vi "Set Page Size.vi"(0 "PDF Report IN":T21(xcontrol), 2 "Page setup":T22={"Page Size"=1, "Orientation"=enum."Portrait", "Custom Layout"={"Width"=0.0, "Height"=0.0}, "Margins"={"Left"=25.0, "Right"=25.0, "Top"=25.0, "Bottom"=25.0}} {"Page Size" items=["Custom", "LETTER", "NOTE", "LEGAL", "TABLOID", "EXECUTIVE", "POSTCARD", "A0", "A1", "A2", "A3", "A4", "A5", "A6", "A7", "A8", "A9", "A10", "B0", "B1", "B2", "B3", "B4", "B5", "B6", "B7", "B8", "B9", "B10", "ARCH_E", "ARCH_D", "ARCH_C", "ARCH_B", "ARCH_A", "FLSA", "FLSE", "HALFLETTER", "_11X17", "ID_1", "ID_2", "ID_3", "LEDGER", "CROWN_QUARTO", "LARGE_CROWN_QUARTO", "DEMY_QUARTO", "ROYAL_QUARTO", "CROWN_OCTAVO", "LARGE_CROWN_OCTAVO", "DEMY_OCTAVO", "ROYAL_OCTAVO", "SMALL_PAPERBACK", "PENGUIN_SMALL_PAPERBACK", "PENGUIN_LARGE_PAPERBACK"]}, 11 "error in (no error)":errorcluster) -> (4 "PDF Report OUT":T21(xcontrol), 15 "error OUT":errorcluster)   [LabVIEW 2013]
doc: "Creates a page break within the PDF report and change the layout of the new page:\n- Page size;\n- Orientation;\n- Margins (mm or in);\n- Custom layout (if Page size = custom, mm or in);\n\nMinimum page size: 3 points x 3 points (1.06 mm x 1.06 mm or 0.042 in x 0.042 in)\nMaximum page size: 14400 points x 14400 points (5.08 m x 5.08 m or 200 in x 200 in)\n\n<B>FRANÇAIS</B>\nAjoute un saut de page dans le rapport PDF et change les caractéristiques de la nouvelle page :\n- Format de la page;\n- Orientation;\n- Marges (mm or in);\n- Format personnalisé (si Page size = custom, mm ou in).\n\nDimensions minimales d'une page: 3 points x 3 points (1.06 mm x 1.06 mm or 0.042 in x 0.042 in).\nDimensions maximales d'une page: 14400 points x 14400 points (5.08 m x 5.08 m or 200 in x 200 in).\n\nVersion 1.0\nDeveloped by Jean-Marc Simard\nCopyright © 2010, Exaprom Inc.\nAll rights reserved.\nLicense: BSD\n\nWith iTextSharp 4.1.6 (http://itextsharp.sourceforge.net)\nunder Mozilla Public License Version 1.1\n(http://www.mozilla.org/MPL/MPL-1.1.html)"
uses:
  Controls/Page setup.ctl
  Controls/Page size.ctl
  Controls/Page Orientation.ctl
  Controls/Page Layout Custom.ctl
  Controls/Page margins.ctl
  Controls/PDF Report Xcontrol/PDF Report.xctl
  C:/Users/MaxCorp/Documents/GitHub/TopView/DLL/itextsharp.dll
  DLL/itextsharp.dll
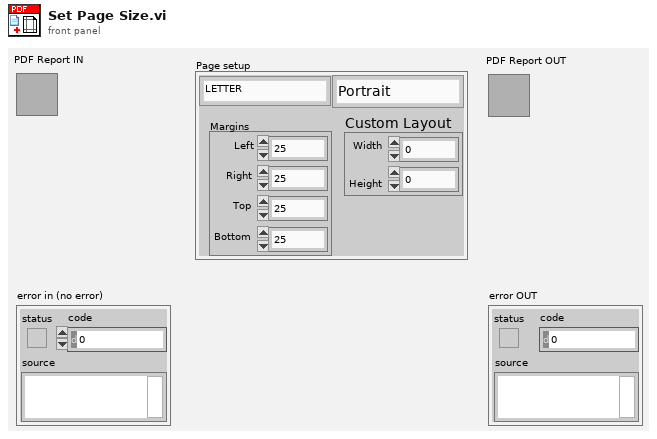
[diagram p1: front panel]
types:
  T1 = typedef "Font cluster.ctl" = cluster{"Name":string, "Size":T2, "Color":T3, "Style":cluster{"Bold":bool, "Italic":bool, "Underline":bool, "Strikeout":bool}}
  T2 = typedef "Font size.ctl" = sgl
  T3 = typedef "Font color.ctl" = u32
  T4 = typedef "Unit.ctl" = enum16{"inch", "mm"}
  T5 = typedef "Paragraphe cluster.ctl" = cluster{" Aligment":T6, "Line spacing":T7}
  T6 = typedef "Texte alignement.ctl" = enum16{"Select", "CENTER", "JUSTIFY", "LEFT", "RIGHT"}
  T7 = typedef "Line spacing.ctl" = enum16{"Select", "1.0", "1.5", "2.0"}
  T8 = typedef "Page dimensions.ctl" = cluster{"Start at page":i32, "Orientation":T9, "widht":sgl, "height":sgl, "Margin left":sgl, "Margin right":sgl, "Margin top":sgl, "Margin bottom":sgl}
  T9 = typedef "Page Orientation.ctl" = enum16{"Portrait", "Landscape"}
  T10 = typedef "Image or Table Caption.ctl" = cluster{"Caption":string, "Separator":string, "Position":enum16{"Above", "Below"}}
  T11 = typedef "Header Footer [ ].ctl" = T12[]
  T12 = typedef "Header Footer cluster.ctl" = cluster{"Start page":i32, "Type":T13, "Alignment":T14, "Vertical Alignement":T15, "Image (%)":sgl, "Page #":T16, "Text":string, "Path":string, "Font":T1, "Font refnum":refnum<k24>, "Line":cluster{"Line":T17, "Thickness (points)":sgl, "Colour":T3}}
  T13 = typedef "Header Footer Type.ctl" = enum16{"Select", "Text", "Text + hyperlink", "Page number", "Image", "Image + hyperlink"}
  T14 = typedef "Header footer horiz alignment.ctl" = enum16{"Left", "Center", "Right"}
  T15 = typedef "Cell Vertical alignment.ctl" = enum16{"TOP", "MIDDLE", "BOTTOM"}
  T16 = typedef "Page number.ctl" = cluster{"Text 1":string, "Text 2":string, "Text 3":string}
  T17 = typedef "Header Footer Line.ctl" = enum16{"No line", "Horizontal line"}
  T18 = typedef "Watermark cluster2.ctl" = cluster{"Show? (F)":bool, "Type":enum16{"Image", "Text"}, "Opacity (%)":sgl, "Rotate(°)":sgl, "Position":cluster{"Position":T19, "X":sgl, "Y":sgl}, "Image path":path, "Scaled(%)":sgl, "Image refnum":refnum<k24>, "Text":string, "Font":cluster{"Name":string, "Size":T2, "Color":T3}, "Font refnum":refnum<k24>, "Alignment":T14, "Automatic":bool}
  T19 = typedef "Watermark Position.ctl" = enum16{"Absolute", "Center (page)", "Center (text section)"}
  T20 = typedef "System Fonts.ctl" = cluster{"Font name [ ]":string[], "Font and file names [ ]":cluster{"Font name":string, "File name":string}[]}
  T21 = cluster{"Document":refnum<k24>, "Writer":refnum<k24>, "Default Font":refnum<k24>, "Default Font cluster":T1, "Path":path, "Unit (default = mm)":T4, "Paragraphe cluster":T5, "Pages dimensions [ ]":T8[], "Captions":cluster{"Image":T10, "Image counter":u16, "Table":T10, "Table counter":u16, "Font":T1}, "Header":T11, "Footer":T11, "Watermark ":T18, "Actual VI name":string, "System Fonts":T20}
  T22 = typedef "Page setup.ctl" = cluster{"Page Size":T23, "Orientation":T9, "Custom Layout":T24, "Margins":T25}
  T23 = typedef "Page size.ctl" = i32
  T24 = typedef "Page Layout Custom.ctl" = cluster{"Width":sgl, "Height":sgl}
  T25 = typedef "Page margins.ctl" = cluster{"Left":sgl, "Right":sgl, "Top":sgl, "Bottom":sgl}
  T26 = cluster{"PageNumber":i32, "Orientation":T9, "Width":sgl, "Height":sgl, "LeftMargin":sgl, "RightMargin":sgl, "TopMargin":sgl, "BottomMargin":sgl}
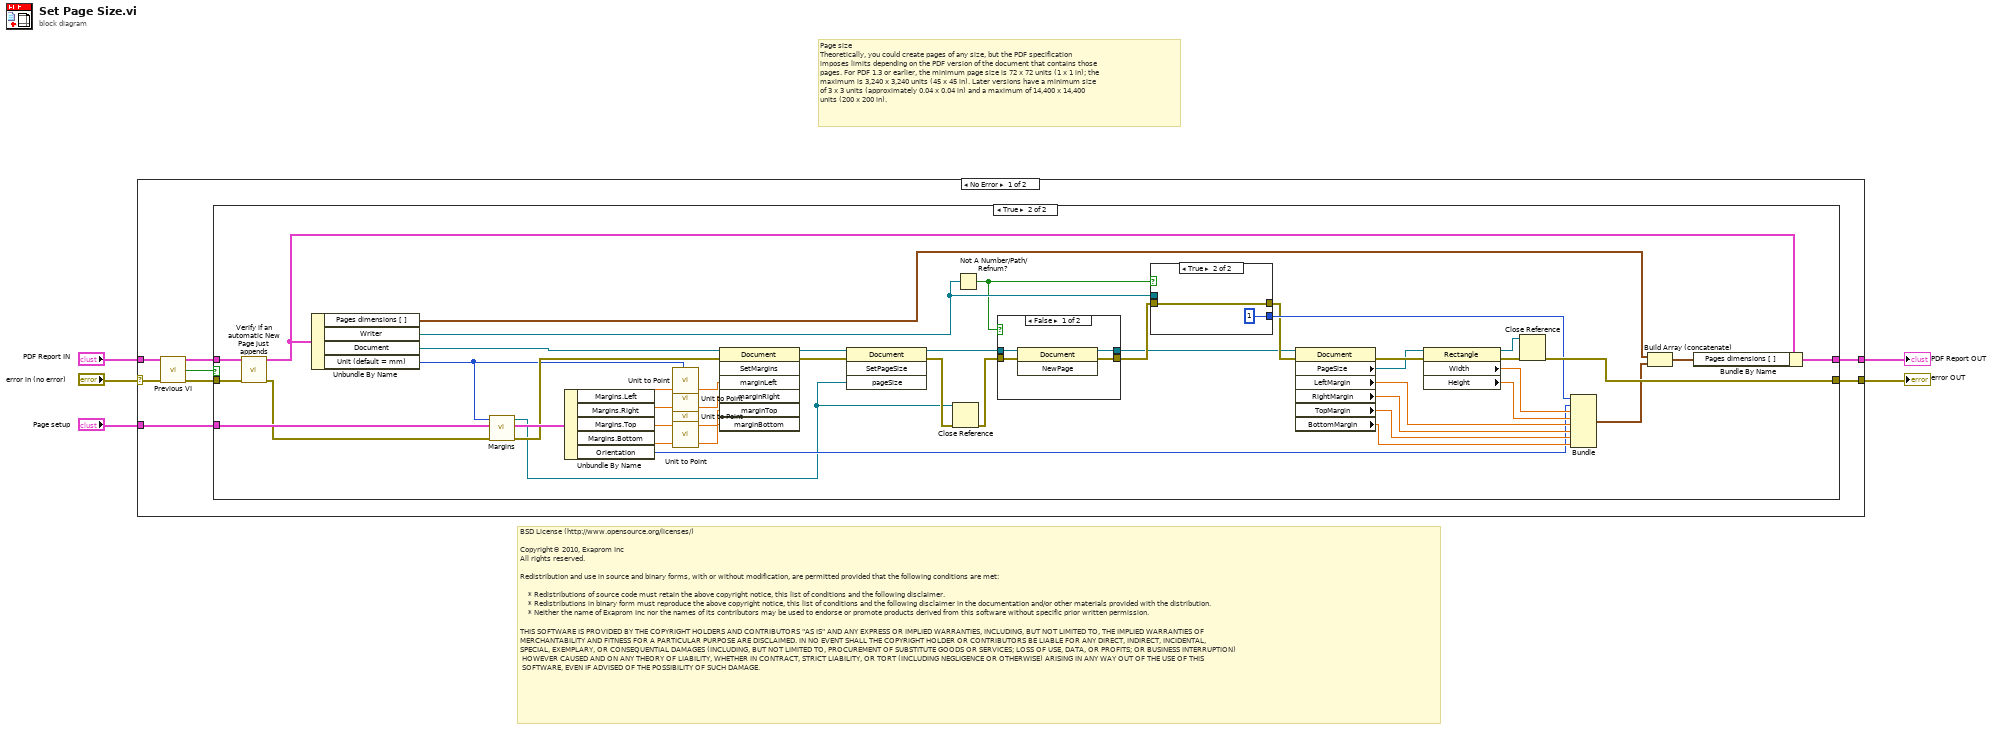
[diagram p0: block diagram]
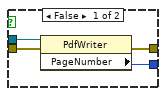
[diagram p4: hidden frame]
diagram:
  # "Page size\nTheoretically, you could create pages of any size, but the PDF specification\nimposes limits depending on the PDF version of the document that contains those\npages. For PDF 1.3 or earlier, the minimum page size is 72 x 72 units (1 x 1 in); the\nmaximum is 3,240 x 3,240 units (45 x 45 in). Later versions have a minimum size\nof 3 x 3 units (approximately 0.04 x 0.04 in) and a maximum of 14,400 x 14,400\nunits (200 x 200 in)."
  # "BSD License (http://www.opensource.org/licenses/)\n\nCopyright© 2010, Exaprom Inc\nAll rights reserved.\n\nRedistribution and use in source and binary forms, with or without modification, are permitted provided that the following conditions are met:\n\n    * Redistributions of source code must retain the above copyright notice, this list of conditions and the following disclaimer.\n    * Redistributions in binary form must reproduce the above copyright notice, this list of conditions and the following disclaimer in the documentation and/or other materials provided with the distribution.\n    * Neither the name of Exaprom Inc nor the names of its contributors may be used to endorse or promote products derived from this software without specific prior written permission.\n\nTHIS SOFTWARE IS PROVIDED BY THE COPYRIGHT HOLDERS AND CONTRIBUTORS \"AS IS\" AND ANY EXPRESS OR IMPLIED WARRANTIES, INCLUDING, BUT NOT LIMITED TO, THE IMPLIED WARRANTIES OF \nMERCHANTABILITY AND FITNESS FOR A PARTICULAR PURPOSE ARE DISCLAIMED. IN NO EVENT SHALL THE COPYRIGHT HOLDER OR CONTRIBUTORS BE LIABLE FOR ANY DIRECT, INDIRECT, INCIDENTAL,\nSPECIAL, EXEMPLARY, OR CONSEQUENTIAL DAMAGES (INCLUDING, BUT NOT LIMITED TO, PROCUREMENT OF SUBSTITUTE GOODS OR SERVICES; LOSS OF USE, DATA, OR PROFITS; OR BUSINESS INTERRUPTION)\n HOWEVER CAUSED AND ON ANY THEORY OF LIABILITY, WHETHER IN CONTRACT, STRICT LIABILITY, OR TORT (INCLUDING NEGLIGENCE OR OTHERWISE) ARISING IN ANY WAY OUT OF THE USE OF THIS\n SOFTWARE, EVEN IF ADVISED OF THE POSSIBILITY OF SUCH DAMAGE."
  n1 = case shown="No Error" "error in (no error)" {
    selector: "error in (no error)" -> [w9 w74]
    tunnel: [w11 w74] -> w3
    tunnel: "Page setup" -> [w6 _]
    tunnel: [w13 w73] -> w2
    tunnel: "PDF Report IN" -> [w12 w73]
    frame No Error {
      n2 = call "Previous VI.vi"("PDF Report IN"=w12, "error in (no error)"=w9) -> ("PDF Report OUT"=w10:T21, "Execute Actual VI"=w8:bool, "error out"=w7:errorcluster)  [unwired: 11 out]
      n3 = case shown="True" w8 {
        tunnel: w6 -> [_ w60]
        tunnel: [w14 w44] -> w13
        tunnel: [w15 w39] -> w11
        tunnel: w10 -> [w14 w22]
        tunnel: w7 -> [w15 w19]
        frame False {
        }
        frame True {
          n4 = call "Verify if an automatic New Page just appends.vi"("PDF Report IN"=w22, "error in (no error)"=w19) -> ("PDF Report OUT"=w20:T21, "error out"=w18:errorcluster)  [unwired: 12 out]
          n5 = Unbundle By Name(w20) -> ("Pages dimensions [ ]"=w16:T8[], "Writer"=w35:refnum<k24>, "Document"=w34:refnum<k24>, "Unit (default = mm)"=w25:T4)
          n6 = call "Margins.vi"("error in (no error)"=w18, "Page setup IN"=w60, "Unit (default = mm)"=w25) -> ("error out"=w26:errorcluster, "Page setup OUT"=w28:T22, "Rectangle"=w24:refnum<k24>)  [unwired: 6 out]
          n7 = Unbundle By Name(w28) -> ("Margins.Left"=w59:sgl, "Margins.Right"=w58:sgl, "Margins.Top"=w57:sgl, "Margins.Bottom"=w56:sgl, "Orientation"=w27:T9)
          n8 = call "Unit to Point.vi"("X unit"=w59, "Unit (default = mm)"=w25) -> ("X point"=w52:sgl)  [unwired: 7 out]
          n9 = call "Unit to Point.vi"("X unit"=w58, "Unit (default = mm)"=w25) -> ("X point"=w53:sgl)  [unwired: 7 out]
          n10 = call "Unit to Point.vi"("X unit"=w57, "Unit (default = mm)"=w25) -> ("X point"=w54:sgl)  [unwired: 7 out]
          n11 = call "Unit to Point.vi"("X unit"=w56, "Unit (default = mm)"=w25) -> ("X point"=w55:sgl)  [unwired: 7 out]
          n12 = invoke class="Document" method="SetMargins"(reference=w34, error in=w26, "marginLeft"=w52, "marginRight"=w53, "marginTop"=w54, "marginBottom"=w55) -> (reference out=w33:refnum<k24>, error out=w21:errorcluster)  [unwired: 1 in, 5 out]
          n13 = invoke class="Document" method="SetPageSize"(reference=w33, error in=w21, "pageSize"=w24) -> (reference out=w32:refnum<k24>, error out=w43:errorcluster)  [unwired: 1 in, 2 out]
          n14 = Close Reference(reference=w24, error in (no error)=w43) -> (error out=w31:errorcluster)
          n15 = Not A Number/Path/Refnum?(number/path/refnum=w35) -> (NaN/Path/Refnum?=w29:bool)
          n16 = case shown="False" w29 {
            tunnel: [w64 w66] -> w17
            tunnel: [w63 w65] -> w30
            tunnel: w31 -> [w62 w65]
            tunnel: w32 -> [w61 w66]
            frame False {
              n17 = invoke class="Document" method="NewPage"(reference=w61, error in=w62) -> (reference out=w64:refnum<k24>, error out=w63:errorcluster)  [unwired: 1 in, 1 out]
            }
            frame True {
            }
          }
          n18 = case shown="True" w29 {
            tunnel: [w69 1 ("PageNumber")] -> w37
            tunnel: w35 -> [w70 _]
            tunnel: w30 -> [w68 w71]
            tunnel: [w67 w71] -> w36
            frame False {
              n19 = property class="PdfWriter"(reference=w70, error in=w68) -> (error out=w67:errorcluster, "PageNumber"=w69:i32)  [unwired: 1 out]
            }
            frame True {
            }
          }
          n20 = property class="Document"(reference=w17, error in=w36) -> (error out=w51:errorcluster, "PageSize"=w23:refnum<k24>, "LeftMargin"=w48:sgl, "RightMargin"=w47:sgl, "TopMargin"=w46:sgl, "BottomMargin"=w45:sgl)  [unwired: 1 out]
          n21 = property class="Rectangle"(reference=w23, error in=w51) -> (reference out=w41:refnum<k24>, error out=w42:errorcluster, "Width"=w50:sgl, "Height"=w49:sgl)
          n22 = Close Reference(reference=w41, error in (no error)=w42) -> (error out=w39:errorcluster)
          n23 = Bundle("PageNumber"=w37, "Orientation"=w27, "Width"=w50, "Height"=w49, "LeftMargin"=w48, "RightMargin"=w47, "TopMargin"=w46, "BottomMargin"=w45) -> (w38:T26)  [unwired: 1 out]
          n24 = Build Array (concatenate)(w16, w38) -> (w40:T8[])
          n25 = Bundle By Name(cluster=w20, "Pages dimensions [ ]"=w40) -> (w44:T21)
        }
      }
    }
    frame Error {
    }
  }
  "error OUT" <- w3
  "PDF Report OUT" <- w2
